vi "CMD_Shoot.vi"(1 "Line":string) -> (0 "Done":bool)   [LabVIEW 2016]
uses:
  Apple Gyro/Apple Pi Gyro Library.lvlib
  Robot Global Data.vi
panel:
  in  "Parameters":i32[](array[numeric])=[1]
  in  "Subcommands":string[](array[string])=["test"]
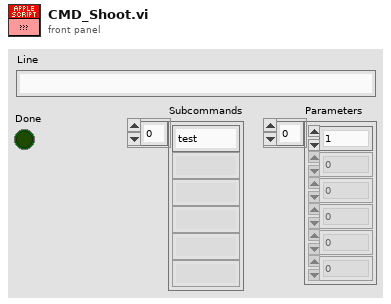
[diagram p1: front panel]
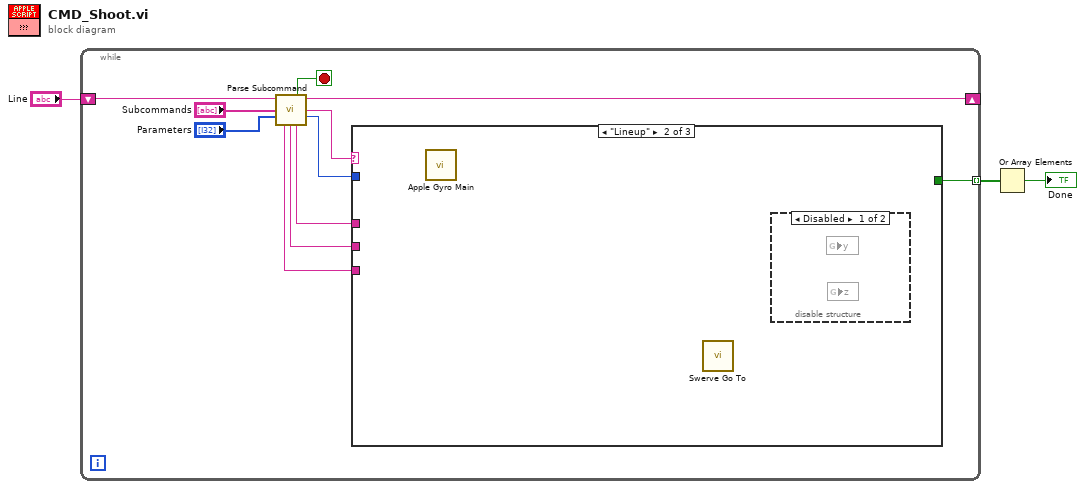
[diagram p0: block diagram]
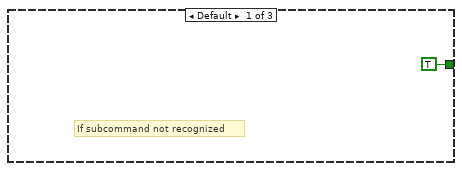
[diagram p2: hidden frame]
diagram:
  n1 = while {
    shift-right: [w11] -> _
    shift-left: "Line" -> [w14]
    tunnel: [w4] -> w2 mode=indexing
    stop <- w10 stop-if-true
    n2 = call "Parse Subcommand.vi"("Text In"=w14, "Subcommands"="Subcommands", "Parameters"="Parameters") -> ("Done"=w10:bool, "Text Out"=w11:string, "Subcommand"=w9:string, "# of Parameters"=w8:i32, "Parameter 3"=w5:string, "Parameter 2"=w6:string, "Parameter 1"=w7:string)  [unwired: 6 in]
    n3 = case shown="\"Lineup\"" w9 {
      tunnel: w8 -> [_ _ _]
      tunnel: w7 -> [_ _ _]
      tunnel: w6 -> [_ _ _]
      tunnel: w5 -> [_ _ _]
      tunnel: [TRUE _ _] -> w4
      frame Default {
        # "If subcommand not recognized"
      }
      frame "Lineup" {
        n4 = call "Apple Gyro Main.vi"() -> ()  [unwired: 4 in, 1 out]
        n5 = call "Swerve Go To.vi"() -> ()  [unwired: 7 in, 1 out]
        n6 = disable-structure shown="Disabled" {
          frame Disabled {
            n7 = global read "Robot Global Data.vi" "y"() -> ()  [unwired: 1 in]
            n8 = global read "Robot Global Data.vi" "z"() -> ()  [unwired: 1 in]
          }
          frame Enabled {
          }
        }
      }
      frame "Shoot" {
      }
    }
  }
  n9 = Or Array Elements(Boolean array=w2) -> (logical OR=→"Done":bool)
